vi "Save Test Config File.vi"(7 "Test Parameters":T1={"Test Name"="Unique Test Name", "Target"=enum."cRIO-9012", "Host IP Address"="0.0.0.0", "Target IP Address"="0.0.0.0", "Shared Variable Host"=enum."Target", "Shared Variable Writer"=enum."Target", "Variable Data Type"=enum."Double", "# of Variables per Library"=1, "Update Rate (Hz)"=1.0, "Read Rate (Hz)"=500.0, "Floor"=5000, "Ceiling"=500, "Delta"=500} {"# of Variables per Library" items=["50"=50, "100"=100, "150"=150, "200"=200, "250"=250, "300"=300, "350"=350, "400"=400, "450"=450, "500"=500]; "Delta" min=50 max=1000000 step=50; "Ceiling" min=50 max=1000000 step=50; "Floor" min=50 max=1000000 step=50}, 8 "error in (no error)":errorcluster, 11 "Root Path":path) -> (0 "error out":errorcluster)   [LabVIEW 2015]
doc: "Save the test configuraiton as an XML file to the test directory."
uses:
  Type Defs/Sequence Parameters.ctl
  Type Defs/Target Type.ctl
  Type Defs/Variable Data Type.ctl
  <vilib>/Utility/xml.llb/Write to XML File(string).vi
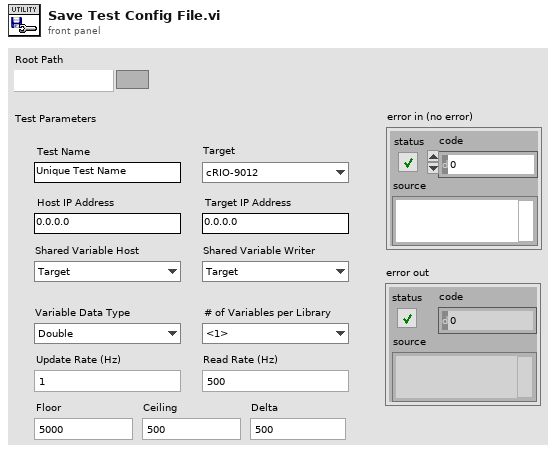
[diagram p1: front panel]
types:
  T1 = typedef "Sequence Parameters.ctl" = cluster{"Test Name":string, "Target":T2, "Host IP Address":string, "Target IP Address":string, "Shared Variable Host":enum16{"Target", "Host"}, "Shared Variable Writer":enum16{"Target", "Host"}, "Variable Data Type":T3, "# of Variables per Library":u16, "Update Rate (Hz)":dbl, "Read Rate (Hz)":dbl, "Floor":u32, "Ceiling":u32, "Delta":u32}
  T2 = typedef "Target Type.ctl" = enum16{"cRIO-9012", "cRIO-9014", "cRIO-9022", "cRIO-9023", "cRIO-9024", "cRIO-9025", "cRIO-9068", "cRIO-9073", "cRIO-9074", "cRIO-9075", "cRIO-9076", "cRIO-9081", "cRIO-9082", "myRIO-1900", "myRIO-1950", "PXI-8101", "PXI-8115", "PXI-8119", "PXI-8820", "PXIe-8100", "PXIe-8101", "PXIe-8133", "PXIe-8135", "PXIe-8820", "sbRIO-9605", "sbRIO-9606", "sbRIO-9623", "sbRIO-9626", "sbRIO-9633", "sbRIO-9636", "Unlisted (Linux-RT)", "Unlisted (PharLap)", "Unlisted (VxWorks)", "Windows Target"}
  T3 = typedef "Variable Data Type.ctl" = enum16{"U8", "U16", "U32", "U64", "I8", "I16", "I32", "I64", "Single", "Double", "Boolean", "String"}
  T4 = enum16{"open", "replace", "create", "open or create", "replace or create", "replace or create with confirmation"}
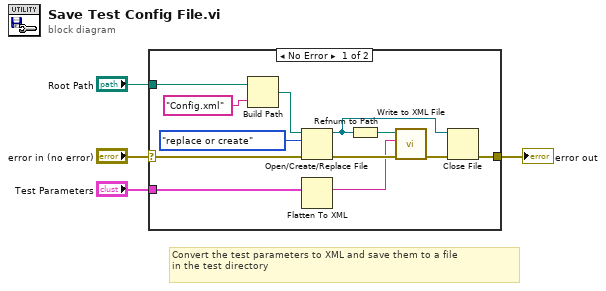
[diagram p0: block diagram]
diagram:
  # "Convert the test parameters to XML and save them to a file\nin the test directory"
  n1 = case shown="No Error" "error in (no error)" {
    selector: "error in (no error)" -> [w14 w17]
    tunnel: "Root Path" -> [w16 _]
    tunnel: "Test Parameters" -> [w10 _]
    tunnel: [w5 w17] -> w1
    frame No Error {
      n2 = Build Path(base path=w16, name or relative path="Config.xml") -> (appended path=w12:path)
      n3 = Open/Create/Replace File(file path (use dialog)=w12, error in=w14, operation (0:open)=T4."replace or create") -> (refnum out=w7:refnum<file>, error out=w11:errorcluster)  [unwired: 3 in, 1 out]
      n4 = Flatten To XML(anything=w10) -> (xml string=w8:string)
      n5 = Refnum to Path(1:w7) -> (0:w9:path)
      n6 = call-poly <vilib>:"Write to XML File.vi"("error in (no error)"=w11, "XML Input"=w8, "XML File Path"=w9) -> ("error out"=w6:errorcluster)  [unwired: 6 in, 2 out]
      n7 = Close File(refnum=w7, error in=w6) -> (error out=w5:errorcluster)  [unwired: 1 out]
    }
    frame Error {
    }
  }
  "error out" <- w1
